vi "Real Dot Product.vi"(2 "Y Vector":dbl[](array[numeric]) format="%.2f", 3 "X Vector":dbl[](array[numeric]) format="%.2f") -> (0 "error":i32, 1 "X * Y":dbl format="%.2f")   [LabVIEW 2013, in "NI_AALBase.lvlib"]
doc: "Computes the dot product of <B>X Vector</B> and <B>Y Vector</B>. The data types you wire to the <B>X Vector</B> and <B>Y Vector</B> inputs determine the polymorphic instance to use."
uses:
  NI_AALBase.lvlib
  lvanlys.dll
panel:
  # "Dot Product"
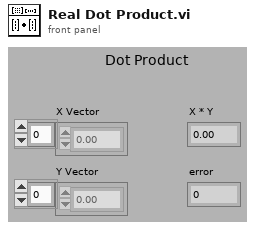
[diagram p1: front panel]
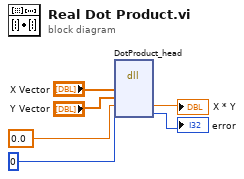
[diagram p0: block diagram]
diagram:
  n1 = dll-call lib="C:/Program Files (x86)/National Instruments/LabVIEW 2013/resource/lvanlys.*" fn="DotProduct_head"("X Vector"="X Vector", "Y Vector"="Y Vector", 0.0, 0) -> (→"X * Y":dbl, →"error":i32)  [unwired: 6 in, 2 out]
